vi "State Logger.vi"() -> ()   [LabVIEW 2011, in "Messenging.lvlib" / "State Logger.lvclass"]
uses:
  State Logger.lvclass
  Interprocess Messenger/TextVarientMessage/MSG.lvclass
  Parallel Process.lvclass
  Interprocess Messenger/TextVarientMessage/Write (no data).vi
  Interprocess Messenger/EventMessenger/EventMessenger.lvclass
  Messsage Logger/MessageLoggerMessage/MessageLoggerMessage.lvclass
  <vilib>/Utility/error.llb/DialogType.ctl
  Messsage Logger/Message Logger.lvclass
  Interprocess Messenger/Send/Send.lvclass
panel:
  in  "Displayed Process":i32(listbox) caption="Sent By:"
  in  "Startup Message":refnum<class "MSG.lvclass">
  out "Table":string[][](table)
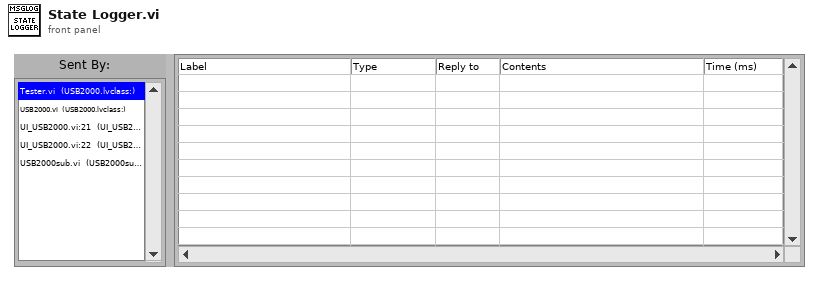
[diagram p1: front panel]
types:
  T1 = enum32{"invalid app kind", "Development System", "Run Time System", "Student Edition", "Embedded LabVIEW", "Evaluation", "Custom"}
  T2 = enum32{"Invalid", "Standard", "Closed", "Hidden", "Minimized", "Maximized"}
  T3 = cluster{"Core":cluster{"Current VI Reference":refnum<vi>, "Close Panel on Exit?":bool}, "New":cluster{"Message":refnum<class "MSG.lvclass">, "MessageTime":u32, "ProcessIndex":i32}, "事件注册引用句柄":refnum<event-registration>, "Processes":string[], "States":cluster{"Table":string[][]}[], "T0":u32}
  T4 = typedef "DialogType.ctl" = u16
  T5 = cluster{"Message":refnum<class "MSG.lvclass">, "MessageTime":u32, "ProcessIndex":i32}
  T6 = cluster{"Current VI Reference":refnum<vi>, "Close Panel on Exit?":bool}
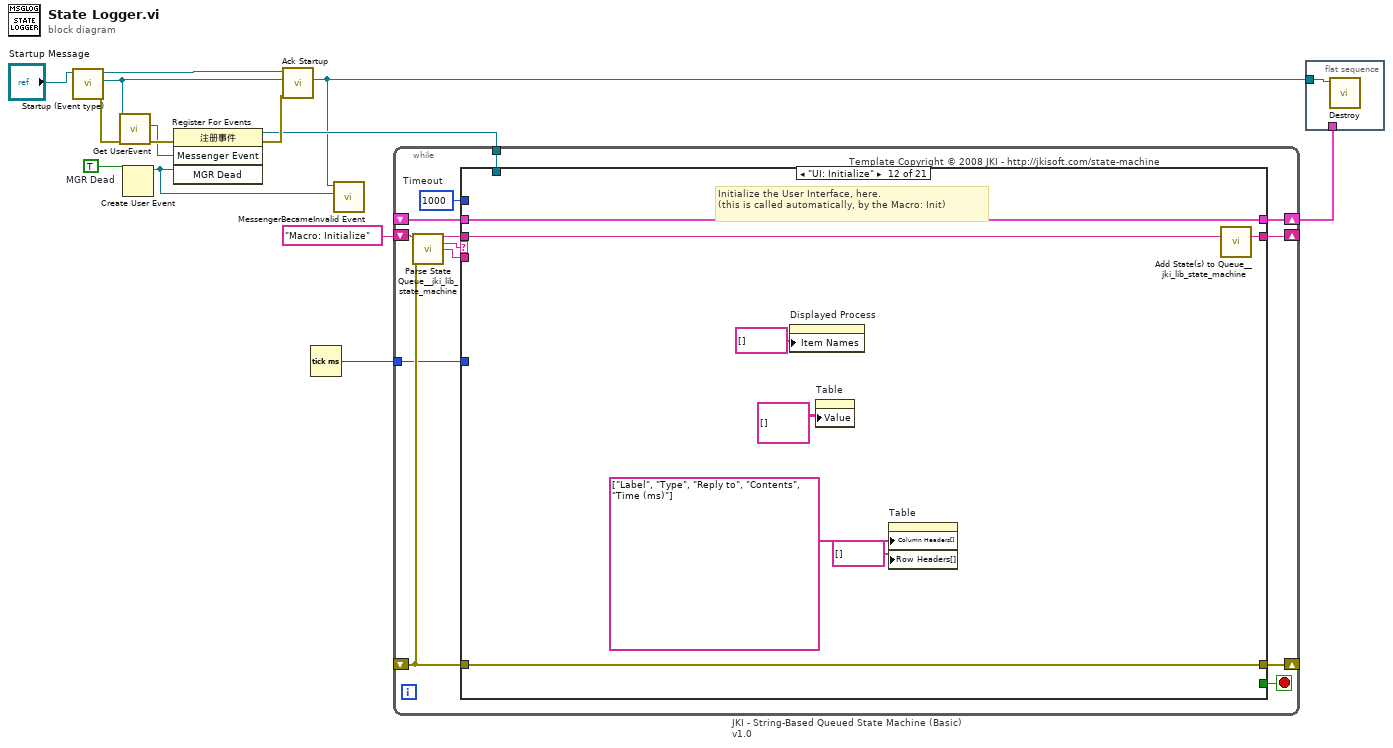
[diagram p0: block diagram]
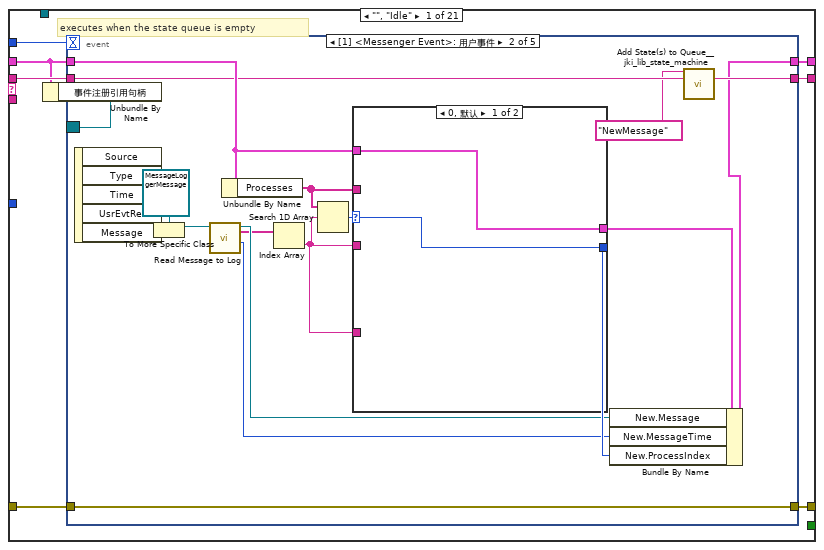
[diagram p2: hidden frame]
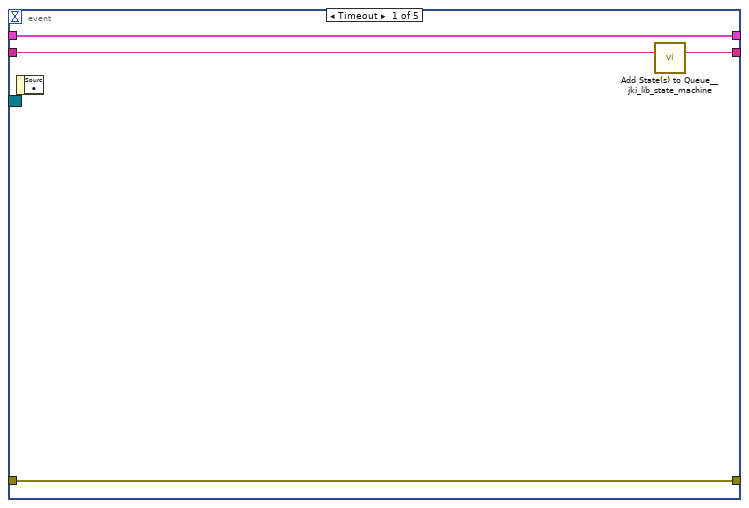
[diagram p3: hidden frame]
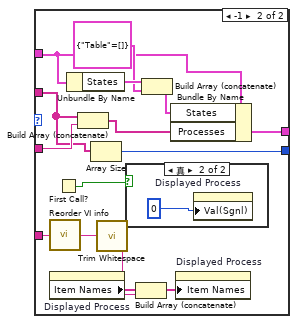
[diagram p4: hidden frame]
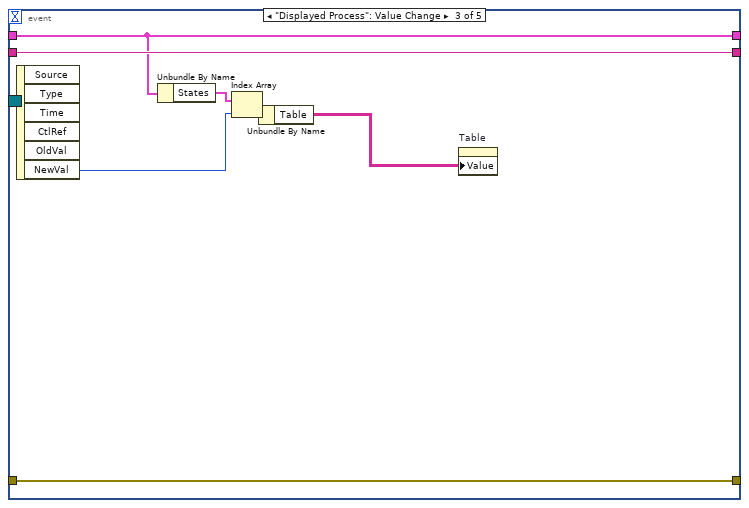
[diagram p6: hidden frame]
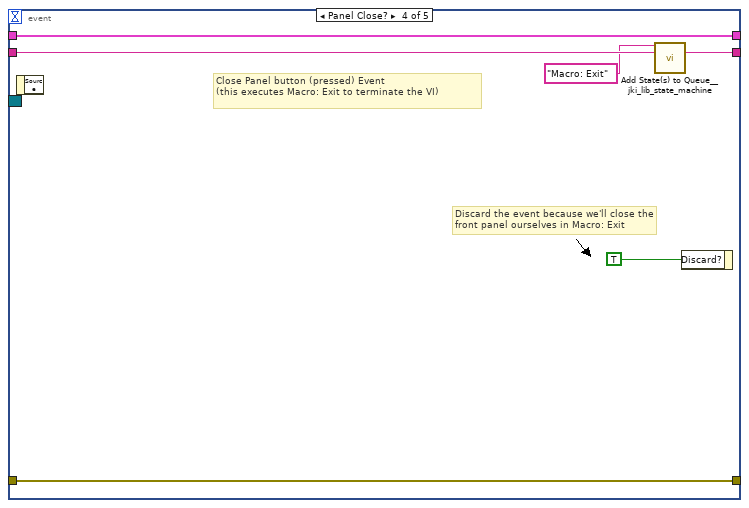
[diagram p7: hidden frame]
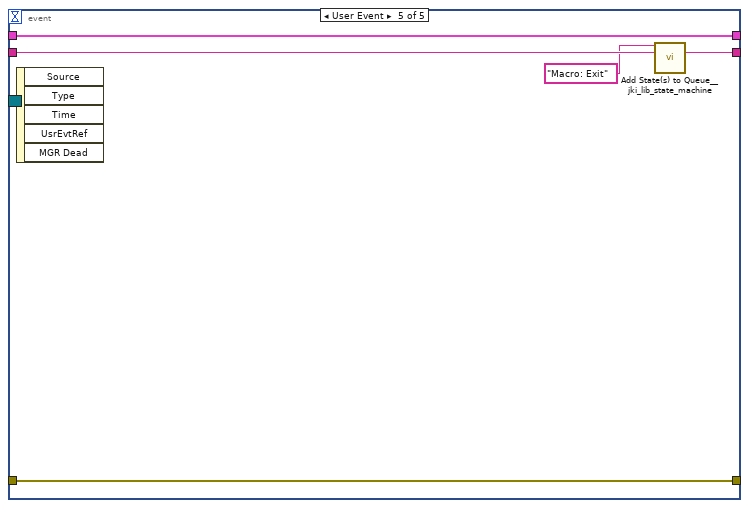
[diagram p8: hidden frame]
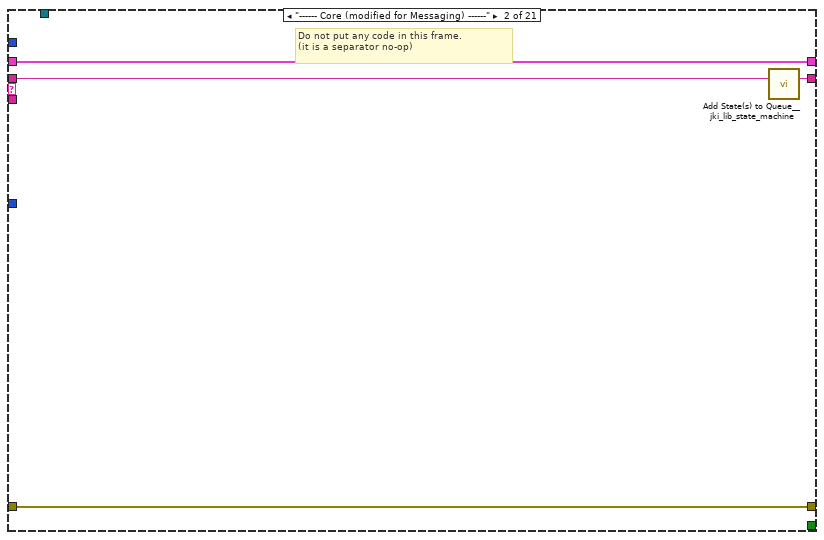
[diagram p9: hidden frame]
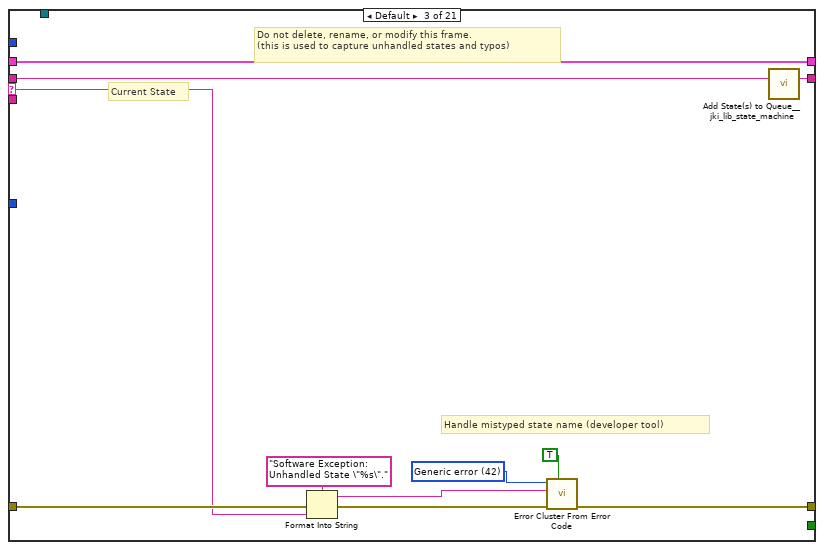
[diagram p10: hidden frame]
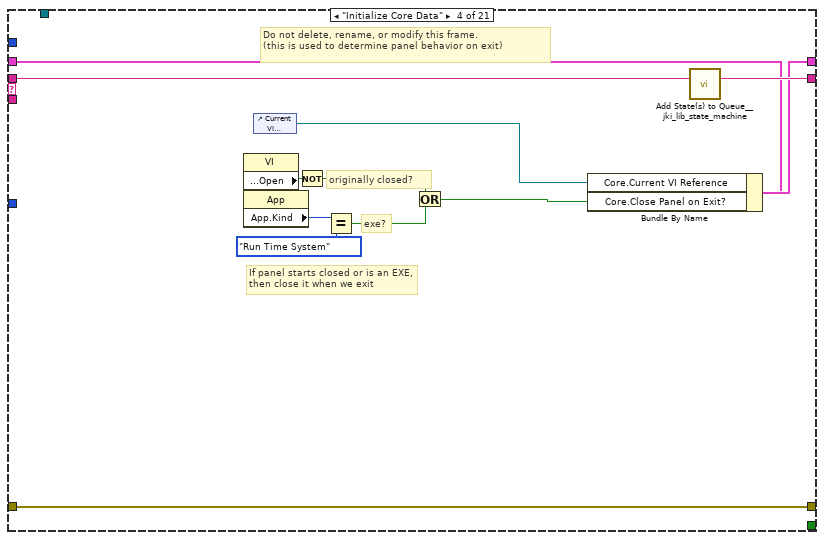
[diagram p11: hidden frame]
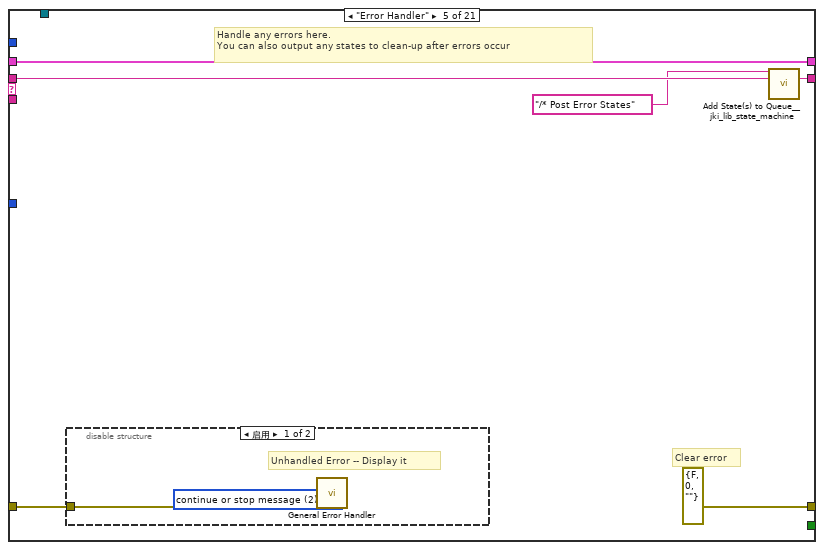
[diagram p12: hidden frame]
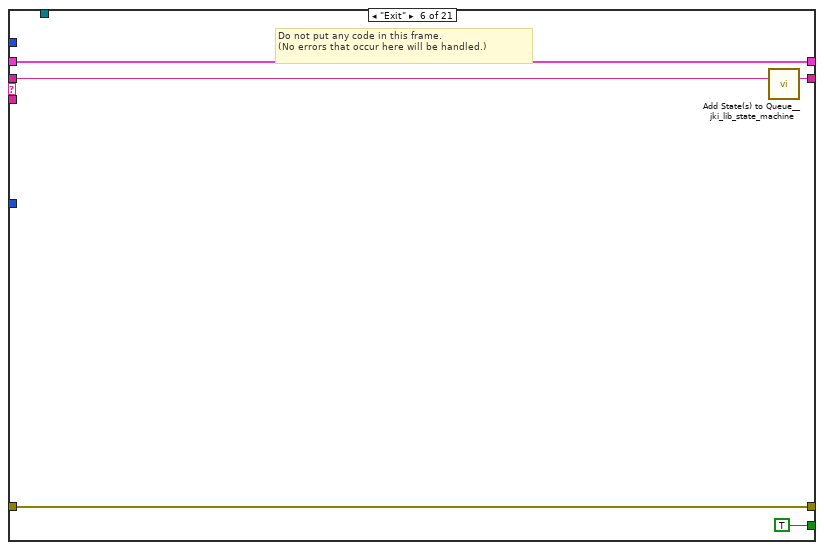
[diagram p14: hidden frame]
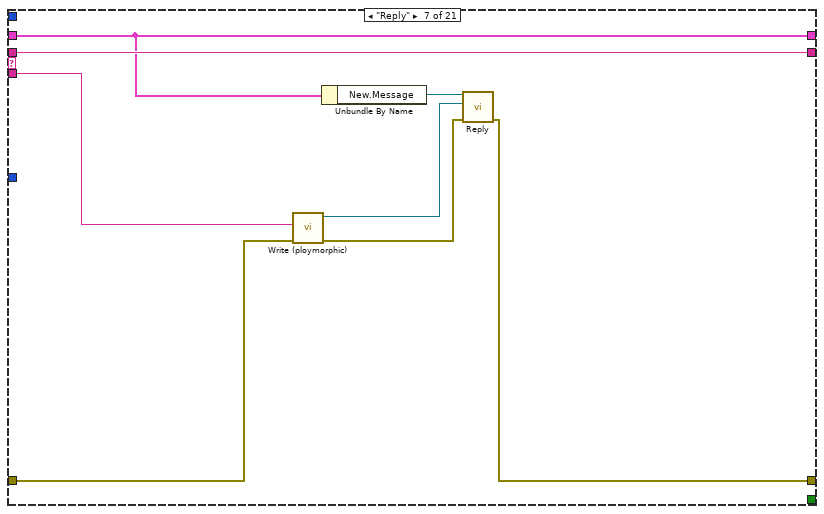
[diagram p15: hidden frame]
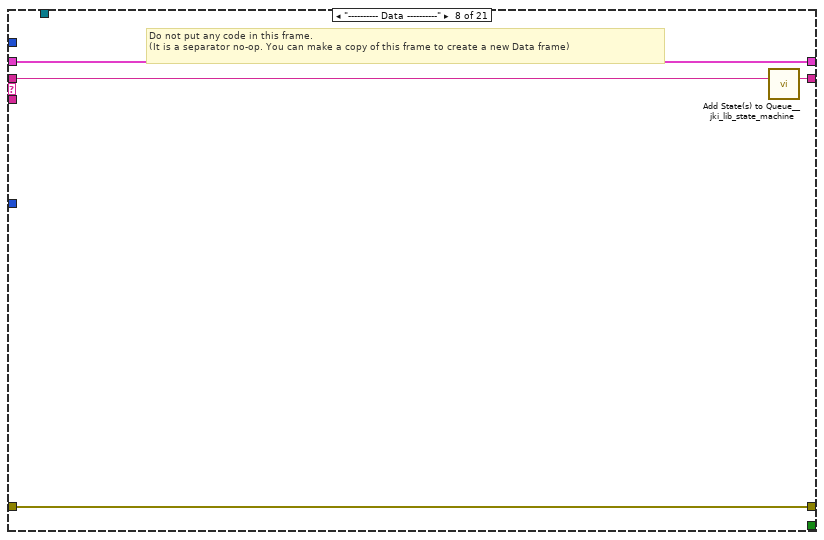
[diagram p16: hidden frame]
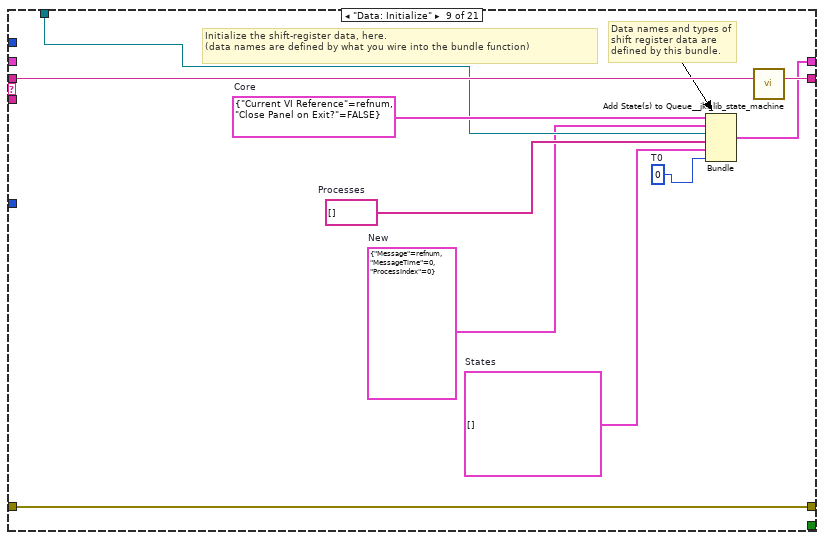
[diagram p17: hidden frame]
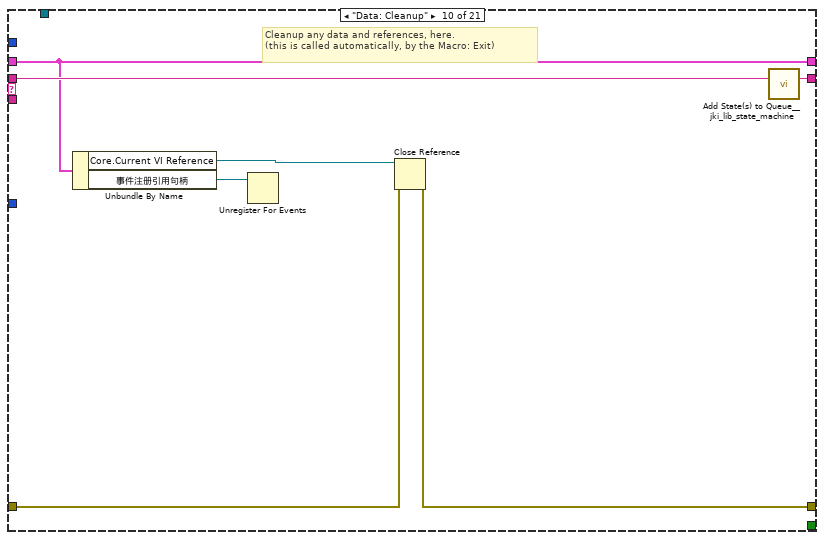
[diagram p18: hidden frame]
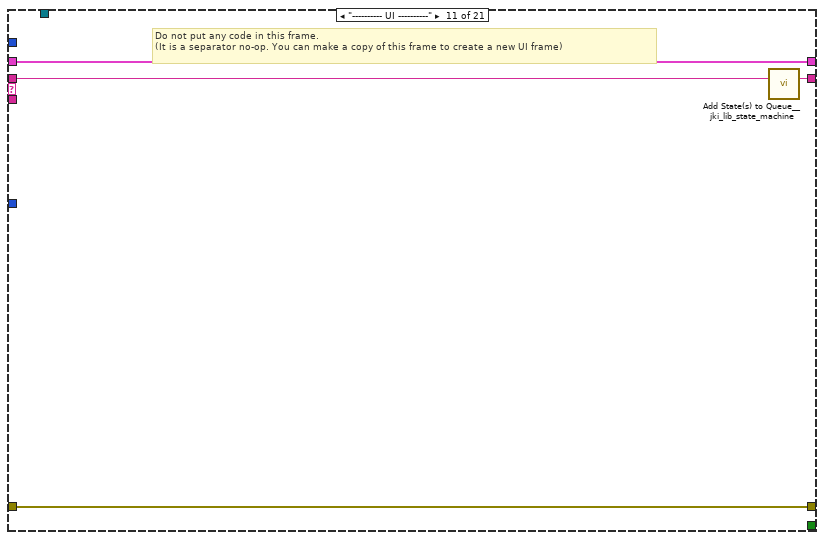
[diagram p19: hidden frame]
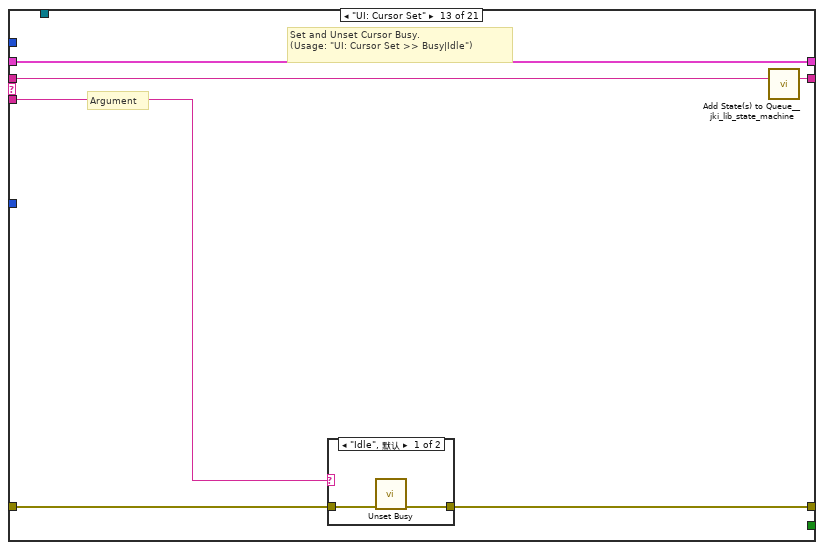
[diagram p20: hidden frame]
diagram:
  w8 = TRUE  # MGR Dead
  n1 = call "Startup (Event type).vi"("Startup Message"="Startup Message") -> ("error out"=w11:errorcluster, "Command Messenger out"=w13:refnum<class "EventMessenger.lvclass">, "Starup Message"=w12:refnum<class "MSG.lvclass">)  [unwired: 2 in, 6 out]
  n2 = call-dynamic "Get UserEvent.vi"("error in"=w11, "EventMessenger"=w13) -> ("error out"=w10:errorcluster, "Messenger Event"=w9:refnum<user-event>)  [unwired: 8 out]
  n3 = Create User Event(user event datatype=w8) -> (user event=w6:refnum<user-event>)  [unwired: 1 in, 1 out]
  n4 = register-events(error in=w10, w9, w6) -> (reference out=w5:refnum<event-registration>, error out=w7:errorcluster)  [unwired: 1 in]
  n5 = call "Ack Startup.vi"("error in"=w7, "Command Messenger"=w13, "Starup Message"=w12) -> ("Command Messenger"=w4:refnum<class "EventMessenger.lvclass">)  [unwired: 3 in, 5 out]
  n6 = Tick Count (ms)() -> (millisecond timer value=w1:u32)
  n7 = call "MessengerBecameInvalid Event.vi"("MGR became Invalid"=w6, "Messenger"=w4) -> ()  [unwired: 1 in, 9 out]
  n8 = while "JKI - String-Based Queued State Machine (Basic) v1.0" {
    shift-right: [w20] -> w3
    shift-left: _ -> [w19]
    shift-right: [w23] -> _
    shift-left: _ -> [w17]
    shift-right: [w22] -> _
    shift-left: "Macro: Initialize" -> [w24]
    tunnel: w5 -> [w16]
    tunnel: w1 -> [w15]
    stop <- w21 stop-if-true
    w18 = 1000  # Timeout
    # "Template Copyright © 2008 JKI - http://jkisoft.com/state-machine"
    n9 = call <vilib>:"Parse State Queue__jki_lib_state_machine.vi"("State Queue"=w24, "Error In (no error)"=w17) -> ("Remaining States"=w26:string, "Current State"=w27:string, "Arguments"=w25:string)  [unwired: 1 in, 10 out]
    n10 = case shown="\"UI: Initialize\"" w27 {
      selector: w27 -> [_ _ w100 _ _ _ _ _ _ _ _ _ _ _ _ _ _ _ _ _ _]
      tunnel: w26 -> [w35 w96 w103 w119 w125 w132 w140 w144 w154 w161 w165 w173 w179 w190 w214 w219 w224 w234 w238 w242 w252]
      tunnel: w25 -> [_ _ _ _ _ _ w133 _ _ _ _ _ w174 w184 _ _ _ _ _ _ _]
      tunnel: w19 -> [w29 w93 w99 w110 w121 w130 w136 w141 _ w156 w162 w171 w177 w186 w213 w216 w220 w225 w235 w241 w248]
      tunnel: [w33 w94 w97 w116 errorcluster {"status"=FALSE, "code"=0, "source"=""} ("error out") w129 w134 w142 w151 w157 w163 w170 w175 w187 w215 w217 w222 w232 w236 w243 w273] -> w23
      tunnel: w17 -> [w32 w94 w104 w116 w120 w129 w135 w142 w151 w158 w163 w170 w176 w188 w215 w217 w222 w232 w236 w243 w273]
      tunnel: [w34 w95 w102 w118 w124 w131 w140 w143 w153 w160 w164 w172 w178 w189 w214 w218 w223 w233 w237 w242 w252] -> w22
      tunnel: [_ _ _ _ _ TRUE _ _ _ _ _ _ _ _ _ _ _ _ _ _ _] -> w21
      tunnel: [w31 w93 w99 w117 w121 w130 w136 w141 w152 w156 w162 w171 w177 w186 w213 w216 w220 w225 w235 w240 w256] -> w20
      tunnel: w18 -> [w30 _ _ _ _ _ _ _ _ _ _ _ _ _ _ _ _ _ _ _ _]
      tunnel: w16 -> [_ _ _ _ _ _ _ _ w149 _ _ _ _ _ _ _ _ _ _ _ _]
      tunnel: w15 -> [_ _ _ _ _ _ _ _ _ _ _ _ _ _ _ _ _ _ _ w239 _]
      frame "", "Idle" {
        # "executes when the state queue is empty"
        n11 = Unbundle By Name(w29) -> ("事件注册引用句柄"=w28:refnum<event-registration>)
        n12 = event shown="[1] <Messenger Event>: 用户事件" {
          selector: w28 -> [_ _ _ _ _]
          dyn-events: _ -> [_ _ _ _ _]
          timeout: w30 -> [_ _ _ _ _]
          tunnel: w35 -> [w39 w49 w81 w87 w92]
          tunnel: [w38 w56 w81 w86 w91] -> w34
          tunnel: w29 -> [w36 w51 w79 w84 w89]
          tunnel: [w37 w52 w80 w85 w90] -> w33
          tunnel: w32 -> [w37 w52 w80 w85 w90]
          tunnel: [w36 w50 w79 w84 w89] -> w31
          event Timeout {
            n13 = event-data() -> ()  [unwired: 2 out]
            n14 = call <vilib>:"Add State(s) to Queue__jki_lib_state_machine.vi"("State(s) in (\"\")"=w39) -> ("States Out"=w38:string)  [unwired: 2 in, 12 out]
          }
          event User Event {
            n15 = event-data() -> ("Message"=w53:refnum<class "MSG.lvclass">)  [unwired: 5 out]
            n16 = To More Specific Class(target class=refnum<class "MessageLoggerMessage.lvclass"> refnum ("Parallel Process.lvlib:MessageLoggerMessage.lvclass"), reference=w53) -> (specific class reference=w55:refnum<class "MessageLoggerMessage.lvclass">)  [unwired: 1 in, 1 out]
            n17 = call "Read Message to Log.vi"("MessageLoggerMessage.lvclass in"=w55) -> ("millisecond timer"=w44:u32, "call chain"=w41:string[], "Messenging.lvlib:Interprocess Message"=w43:refnum<class "MSG.lvclass">)  [unwired: 1 in, 7 out]
            n18 = Unbundle By Name(w51) -> ("Processes"=w46:string[])
            n19 = Index Array(array=w41) -> (element=w40:string)  [unwired: 1 in]
            n20 = Search 1D Array(1D array=w46, element=w40) -> (index of element=w47:i32)  [unwired: 1 out]
            n21 = case shown="0, 默认" w47 {
              selector: w47 -> [w58 _]
              tunnel: [w57 w73] -> w48
              tunnel: w51 -> [w57 w59]
              tunnel: w46 -> [_ w64]
              tunnel: w40 -> [_ w72]
              tunnel: [w58 w70] -> w45
              tunnel: w40 -> [_ w69]
              frame 0, Default {
              }
              frame -1 {
                n22 = call "Reorder VI info.vi"("chain"=w69) -> ("Reorderded"=w65:string)
                n23 = property on="Displayed Process" class="LstBox (严格)"() -> ("Item Names"=w68:string[])  [unwired: 2 in, 2 out]
                n24 = First Call?() -> (First Call?: T/F=w60:bool)
                n25 = Unbundle By Name(w59) -> ("States"=w63:cluster{"Table":string[][]}[])
                n26 = Build Array (concatenate)(w64, w72) -> (w71:string[])
                n27 = Array Size(array=w64) -> (size(s)=w70:i32)
                n28 = call <vilib>:"Trim Whitespace.vi"("string"=w65) -> ("trimmed string"=w66:string)  [unwired: 1 in]
                n29 = case shown="真" w60 {
                  frame False {
                  }
                  frame True {
                    n30 = property on="Displayed Process" class="LstBox (严格)"("Val(Sgnl)"=0 ("Value (Signaling)")) -> ()  [unwired: 2 in, 2 out]
                  }
                }
                n31 = Build Array (concatenate)(w68, w66) -> (w67:string[])
                n32 = Build Array (concatenate)(w63, cluster{"Table":string[][]} {"Table"=[]} ("element")) -> (w61:cluster{"Table":string[][]}[])
                n33 = Bundle By Name(cluster=w59, "States"=w61, "Processes"=w71) -> (w73:T3)
                n34 = property on="Displayed Process" class="LstBox (严格)"("Item Names"=w67) -> ()  [unwired: 2 in, 2 out]
              }
            }
            n35 = Bundle By Name(cluster=w48, "New.Message"=w43, "New.MessageTime"=w44, "New.ProcessIndex"=w45) -> (w50:T3)
            n36 = call <vilib>:"Add State(s) to Queue__jki_lib_state_machine.vi"("State(s) in Front (\"\")"="NewMessage" ("State(s) in Front (\"\")"), "State(s) in (\"\")"=w49) -> ("States Out"=w56:string)  [unwired: 1 in, 12 out]
          }
          event "Displayed Process": Value Change {
            n37 = event-data() -> ("NewVal"=w77:i32)  [unwired: 6 out]
            n38 = Unbundle By Name(w79) -> ("States"=w78:cluster{"Table":string[][]}[])
            n39 = Index Array(array=w78, index=w77) -> (element=w76:cluster{"Table":string[][]})
            n40 = Unbundle By Name(w76) -> ("Table"=w75:string[][])
            n41 = property on="Table" class="Tbl (严格)"("Value"=w75) -> ()  [unwired: 2 in, 2 out]
          }
          event Panel Close? {
            # "Discard the event because we'll close the front panel ourselves in Macro: Exit"
            # "Close Panel button (pressed) Event\n(this executes Macro: Exit to terminate the VI)"
            n42 = event-data() -> ()  [unwired: 2 out]
            n43 = call <vilib>:"Add State(s) to Queue__jki_lib_state_machine.vi"("State(s) in Front (\"\")"="Macro: Exit", "State(s) in (\"\")"=w87) -> ("States Out"=w86:string)  [unwired: 1 in, 12 out]
            n44 = event-data("Discard?"=TRUE) -> ()  [unwired: 1 in, 1 out]
          }
          event User Event {
            n45 = event-data() -> ()  [unwired: 6 out]
            n46 = call <vilib>:"Add State(s) to Queue__jki_lib_state_machine.vi"("State(s) in Front (\"\")"="Macro: Exit", "State(s) in (\"\")"=w92) -> ("States Out"=w91:string)  [unwired: 1 in, 12 out]
          }
        }
      }
      frame "------ Core (modified for Messaging) ------" {
        # "Do not put any code in this frame.\n(it is a separator no-op)"
        n47 = call <vilib>:"Add State(s) to Queue__jki_lib_state_machine.vi"("State(s) in (\"\")"=w96) -> ("States Out"=w95:string)  [unwired: 2 in, 12 out]
      }
      frame Default {
        w106 = 42 items=["No error", "Argument error", "Memory is full", "Out of zone", "End of file", "File already open", "Generic file I/O error", "File not found", "File permission error", "Disk is full", "Duplicate path", "Too many files open", "System feature not enabled", "Resource file not found", "Cannot add resource", "Resource not found", "Image not found", "Image memory error", "Pen does not exist", "Config type invalid", "Config token not found", "Config parse error", "Config memory error", "Bad external code format", "Bad external code offset", "External code not present", "Null window", "Destroy window error", "Null menu", "Print aborted", "Bad print record", "Print driver error", "Windows error during printing", "Memory error during printing", "Print dialog error", "Generic print error", "Invalid device refnum", "Device not found", "Device parameter error", "Device unit error", "Cannot open device", "Device call aborted", "Generic error", "Cancelled by user", "Object ID too low", "Object ID too high", "Object not in heap", "Unknown heap", "Unknown object (invalid DefProc)", "Unknown object (DefProc not in table)", "Message out of range", "Invalid (null) method", "Unknown message", "Manager call not supported", "Bad address", "Network operation in progress", "Network operation timed out", "Connection is busy", "Network attribute not supported", "Network error", "Address in use", "System out of memory", "Connection aborted", "Connection refused", "Not connected", "Already connected", "Connection closed", "Initialization error (interapplication manager)", "Bad occurrence", "Wait on unbound occurrence handler", "Occurrence queue overflow", "Datalog type conflict", "Unused", "Unrecognized type (interapplication manager)", "Memory corrupt", "Failed to make temporary DLL", "Old CIN version", "Drag socket not found", "Failed to load drop-object", "Failed to register OLE object", "Failed to release OLE object", "Format specifier type mismatch", "Unknown format specifier", "Too few format specifiers", "Too many format specifiers", "Scan failed", "Newer CIN version", "Error converting to variant", "Runtime menu error", "Password tampered", "Variant attribute not found", "Incompatible variant data type", "Event data is not available", "Event Store is not present", "Occurrence is not found", "Event Queue is not created", "Event info is not available", "Refnum passed is NULL", "Error retrieving Class GUID", "Error retrieving CoClass GUID", "Error retrieving TypeLib GUID.", "Bad built application magic bytes.", "Specific driver is different from the specific driver associated with the Logical Name.", "There is no session opened to the class driver.", "Max Error", "MAX - Error with config objects", "MAX - Error loading configuration", "MAX - Group not supported"]
        # "Current State"
        # "Do not delete, rename, or modify this frame.\n(this is used to capture unhandled states and typos)"
        # "Handle mistyped state name (developer tool)"
        n48 = Format Into String(format string="Software Exception: Unhandled State \"%s\"." ("message"), error in=w104, w100) -> (resulting string=w98:string, error out=w105:errorcluster)  [unwired: 1 in]
        n49 = call <vilib>:"Error Cluster From Error Code.vi"("show call chain? (False)"=TRUE, "error in (no error)"=w105, "error message (\"\")"=w98, "error code (0)"=w106) -> ("error out"=w97:errorcluster)  [unwired: 5 out]
        n50 = call <vilib>:"Add State(s) to Queue__jki_lib_state_machine.vi"("State(s) in (\"\")"=w103) -> ("States Out"=w102:string)  [unwired: 2 in, 12 out]
      }
      frame "Initialize Core Data" {
        # "Do not delete, rename, or modify this frame.\n(this is used to determine panel behavior on exit)"
        # "originally closed?"
        # "exe?"
        # "If panel starts closed or is an EXE, then close it when we exit"
        n51 = property class="VI"() -> ("Front Panel.Open"=w115:bool)  [unwired: 2 in, 2 out]
        n52 = property class="App"() -> ("App.Kind"=w114:T1)  [unwired: 2 in, 2 out]
        n53 = control-ref of="Current VI Reference"() -> (w108:refnum<vi>)
        n54 = Not(x=w115) -> (.not. x?=w112:bool)
        n55 = Equal?(x=w114, y=T1."Run Time System" ("Application:Kind")) -> (x = y?=w111:bool)
        n56 = Or(x=w112, y=w111) -> (x .or. y?=w109:bool)
        n57 = Bundle By Name(cluster=w110, "Core.Current VI Reference"=w108, "Core.Close Panel on Exit?"=w109) -> (w117:T3)
        n58 = call <vilib>:"Add State(s) to Queue__jki_lib_state_machine.vi"("State(s) in (\"\")"=w119) -> ("States Out"=w118:string)  [unwired: 2 in, 12 out]
      }
      frame "Error Handler" {
        # "Handle any errors here.\nYou can also output any states to clean-up after errors occur"
        # "Clear error"
        n59 = disable-structure shown="启用" {
          disable-tunnel: w120 -> [w127 _]
          frame Enabled {
            w126 = T4 2 items=["no dialog", "OK message", "continue or stop message", "OK message + warnings", "continue/stop + warnings"] ("type of dialog (OK msg:1)")
            # "Unhandled Error -- Display it"
            n60 = call <vilib>:"General Error Handler.vi"("type of dialog (OK msg:1)"=w126, "error in (no error)"=w127) -> ()  [unwired: 14 out]
          }
          frame Disabled {
          }
        }
        n61 = call <vilib>:"Add State(s) to Queue__jki_lib_state_machine.vi"("State(s) in Front (\"\")"="/* Post Error States", "State(s) in (\"\")"=w125) -> ("States Out"=w124:string)  [unwired: 1 in, 12 out]
      }
      frame "Exit" {
        # "Do not put any code in this frame.\n(No errors that occur here will be handled.)"
        n62 = call <vilib>:"Add State(s) to Queue__jki_lib_state_machine.vi"("State(s) in (\"\")"=w132) -> ("States Out"=w131:string)  [unwired: 2 in, 12 out]
      }
      frame "Reply" {
        n63 = call-poly "Write (ploymorphic).vi"("error in (no error)"=w135, "Label"=w133) -> ("error out"=w137:errorcluster, "Message"=w138:refnum<class "MSG.lvclass">)  [unwired: 8 out]
        n64 = Unbundle By Name(w136) -> ("New.Message"=w139:refnum<class "MSG.lvclass">)
        n65 = call-dynamic "Reply.vi"("error in (no error)"=w137, "Reply"=w138, "Message to Reply to"=w139) -> ("error out"=w134:errorcluster)  [unwired: 8 out]
      }
      frame "---------- Data ----------" {
        # "Do not put any code in this frame.\n(It is a separator no-op. You can make a copy of this frame to create a new Data frame)"
        n66 = call <vilib>:"Add State(s) to Queue__jki_lib_state_machine.vi"("State(s) in (\"\")"=w144) -> ("States Out"=w143:string)  [unwired: 2 in, 12 out]
      }
      frame "Data: Initialize" {
        w146 = cluster{"Table":string[][]}[] []  # States
        w147 = T5 {"Message"=refnum, "MessageTime"=0, "ProcessIndex"=0}  # New
        w145 = u32 0  # T0
        w148 = string[] []  # Processes
        w150 = T6 {"Current VI Reference"=refnum, "Close Panel on Exit?"=FALSE}  # Core
        # "Data names and types of shift register data are defined by this bundle."
        # "Initialize the shift-register data, here.\n(data names are defined by what you wire into the bundle function)"
        n67 = Bundle("Core"=w150, "New"=w147, "事件注册引用句柄"=w149, "Processes"=w148, "States"=w146, "T0"=w145) -> (w152:T3)  [unwired: 1 out]
        n68 = call <vilib>:"Add State(s) to Queue__jki_lib_state_machine.vi"("State(s) in (\"\")"=w154) -> ("States Out"=w153:string)  [unwired: 2 in, 12 out]
      }
      frame "Data: Cleanup" {
        # "Cleanup any data and references, here.\n(this is called automatically, by the Macro: Exit)"
        n69 = Unbundle By Name(w156) -> ("Core.Current VI Reference"=w159:refnum<vi>, "事件注册引用句柄"=w155:refnum<event-registration>)
        n70 = Unregister For Events(event registration refnum=w155) -> ()  [unwired: 1 in, 1 out]
        n71 = Close Reference(reference=w159, error in (no error)=w158) -> (error out=w157:errorcluster)
        n72 = call <vilib>:"Add State(s) to Queue__jki_lib_state_machine.vi"("State(s) in (\"\")"=w161) -> ("States Out"=w160:string)  [unwired: 2 in, 12 out]
      }
      frame "---------- UI ----------" {
        # "Do not put any code in this frame.\n(It is a separator no-op. You can make a copy of this frame to create a new UI frame)"
        n73 = call <vilib>:"Add State(s) to Queue__jki_lib_state_machine.vi"("State(s) in (\"\")"=w165) -> ("States Out"=w164:string)  [unwired: 2 in, 12 out]
      }
      frame "UI: Initialize" {
        # "Initialize the User Interface, here.\n(this is called automatically, by the Macro: Init)"
        n74 = property on="Displayed Process" class="LstBox (严格)"("Item Names"=string[] []) -> ()  [unwired: 2 in, 2 out]
        n75 = property on="Table" class="Tbl (严格)"("Value"=string[][] [] ("Table")) -> ()  [unwired: 2 in, 2 out]
        n76 = property on="Table" class="Tbl (严格)"("Column Headers[]"=string[] ["Label", "Type", "Reply to", "Contents", "Time (ms)"] ("Row Header Strings[]"), "Row Headers[]"=string[] [] ("Row Header Strings[]")) -> ()  [unwired: 2 in, 2 out]
        n77 = call <vilib>:"Add State(s) to Queue__jki_lib_state_machine.vi"("State(s) in (\"\")"=w173) -> ("States Out"=w172:string)  [unwired: 2 in, 12 out]
      }
      frame "UI: Cursor Set" {
        # "Argument"
        # "Set and Unset Cursor Busy.\n(Usage: \"UI: Cursor Set >> Busy|Idle\")"
        n78 = case shown="\"Idle\", 默认" w174 {
          tunnel: w176 -> [w181 w183]
          tunnel: [w180 w182] -> w175
          frame "Idle", Default {
            n79 = call <vilib>:"Unset Busy.vi"("error in (no error)"=w181) -> ("error out"=w180:errorcluster)  [unwired: 1 in, 9 out]
          }
          frame "Busy" {
            n80 = call <vilib>:"Set Busy.vi"("error in (no error)"=w183) -> ("error out"=w182:errorcluster)  [unwired: 3 in, 7 out]
          }
        }
        n81 = call <vilib>:"Add State(s) to Queue__jki_lib_state_machine.vi"("State(s) in (\"\")"=w179) -> ("States Out"=w178:string)  [unwired: 2 in, 12 out]
      }
      frame "UI: Front Panel State" {
        # "Argument"
        # "Set Front Panel Open or Closed\n(Usage: \"UI: Front Panel State >> Open|Close\")"
        n82 = Unbundle By Name(w186) -> ("Core.Current VI Reference"=w185:refnum<vi>)
        n83 = case shown="\"Open\", 默认" w184 {
          tunnel: w188 -> [w194 w207]
          tunnel: [w196 w208] -> w187
          tunnel: w185 -> [w195 w205]
          frame "Open", Default {
            n84 = property class="VI"(reference=w195, error in=w194) -> (reference out=w192:refnum<vi>, error out=w193:errorcluster, "Front Panel.Open"=w191:bool)
            n85 = case shown="假" w191 {
              tunnel: [w199 w202] -> w196
              tunnel: w193 -> [w198 w202]
              tunnel: w192 -> [w197 _]
              frame False {
                n86 = invoke class="VI" method="FP.Open"(reference=w197, error in=w198, "Activate"=TRUE, "State"=T2."Standard") -> (error out=w199:errorcluster)  [unwired: 1 in, 4 out]
              }
              frame True {
              }
            }
          }
          frame "Close" {
            n87 = property class="VI"(reference=w205, error in=w207) -> (reference out=w204:refnum<vi>, error out=w206:errorcluster, "Front Panel.Open"=w203:bool)
            n88 = case shown="真" w203 {
              tunnel: [w209 w212] -> w208
              tunnel: w206 -> [w209 w211]
              tunnel: w204 -> [_ w210]
              frame False {
              }
              frame True {
                n89 = invoke class="VI" method="FP.Close"(reference=w210, error in=w211) -> (error out=w212:errorcluster)  [unwired: 1 in, 2 out]
              }
            }
          }
        }
        n90 = call <vilib>:"Add State(s) to Queue__jki_lib_state_machine.vi"("State(s) in (\"\")"=w190) -> ("States Out"=w189:string)  [unwired: 2 in, 12 out]
      }
      frame "UI: ProcessSelect" {
        n91 = Unbundle By Name(w213) -> ()  [unwired: 1 out]
      }
      frame "---------- Macro ----------" {
        # "Do not put any code in this frame.\n(It is a separator no-op. You can make a copy of this frame to create a new Macro frame)"
        n92 = call <vilib>:"Add State(s) to Queue__jki_lib_state_machine.vi"("State(s) in (\"\")"=w219) -> ("States Out"=w218:string)  [unwired: 2 in, 12 out]
      }
      frame "Macro: Initialize" {
        w221 = "Data: Initialize\nInitialize Core Data\nUI: Initialize\nInitialize\n// UI: Front Panel State >> Open"  # Data: Initialize Initialize Core Data UI: Initialize Initialize // UI: Front Panel State >> Open
        # "Initialization Macro\n(This is called once, when the VI starts)"
        n93 = call <vilib>:"Add State(s) to Queue__jki_lib_state_machine.vi"("State(s) in Front (\"\")"=w221, "State(s) in (\"\")"=w224) -> ("States Out"=w223:string)  [unwired: 1 in, 12 out]
      }
      frame "Macro: Exit" {
        # "Exit Macro\n(This is called once, when the VI exits)"
        n94 = Unbundle By Name(w225) -> ("Core.Close Panel on Exit?"=w231:bool)
        n95 = Select(t="//UI: Front Panel State >> Close", s=w231, f="") -> (s? t:f=w228:string)
        n96 = call <vilib>:"Add State(s) to Queue__jki_lib_state_machine.vi"("State(s) in (\"\")"=w228, "State(s) at Back (\"\")"="\nData: Cleanup\nExit") -> ("States Out"=w226:string)  [unwired: 1 in, 12 out]
        n97 = call <vilib>:"Add State(s) to Queue__jki_lib_state_machine.vi"("State(s) in Front (\"\")"=w226, "State(s) in (\"\")"=w234) -> ("States Out"=w233:string)  [unwired: 1 in, 12 out]
      }
      frame "---------- New Category ----------" {
        # "Template Separator\n(You can make a copy of, or modify, this frame)"
        n98 = call <vilib>:"Add State(s) to Queue__jki_lib_state_machine.vi"("State(s) in (\"\")"=w238) -> ("States Out"=w237:string)  [unwired: 2 in, 12 out]
      }
      frame "Initialize" {
        n99 = Bundle By Name(cluster=w241, "T0"=w239) -> (w240:T3)
      }
      frame "NewMessage" {
        n100 = Unbundle By Name(w248) -> ("States"=w259:cluster{"Table":string[][]}[], "New.ProcessIndex"=w253:i32)
        n101 = Unbundle By Name(w248) -> ("New.Message"=w265:refnum<class "MSG.lvclass">)
        n102 = Unbundle By Name(w248) -> ("New.MessageTime"=w247:u32, "T0"=w244:u32)
        n103 = call-dynamic "Read Label.vi"("Message"=w265) -> ("Label"=w264:string, "Message"=w266:refnum<class "MSG.lvclass">)  [unwired: 1 in, 8 out]
        n104 = Index Array(array=w259, index=w253) -> (element=w258:cluster{"Table":string[][]})
        n105 = Equal?(x="Displayed Process", y=w253) -> (x = y?=w251:bool)
        n106 = call-dynamic "Read Reply Messenger.vi"("Messege"=w266) -> ("Reply to..."=w271:refnum<class "Send.lvclass">, "Message"=w270:refnum<class "MSG.lvclass">)  [unwired: 1 in, 8 out]
        n107 = Unbundle By Name(w258) -> ("Table"=w260:string[][])
        n108 = Subtract(x=w247, y=w244) -> (x-y=w245:u32)
        n109 = call-dynamic "Message Class.vi"("Message"=w270) -> ("Message Class"=w267:string, "Message"=w268:refnum<class "MSG.lvclass">)  [unwired: 1 in, 8 out]
        n110 = call-dynamic "Text Description.vi"("Send in"=w271) -> ("Description"=w272:string)  [unwired: 10 out]
        n111 = Index Array(array=w260, index (col)=0 ("index (row)")) -> (element=w261:string[])  [unwired: 1 in]
        n112 = call-dynamic "Contents Summary Text.vi"("Message"=w268) -> ("Contents Summary Text"=w269:string)  [unwired: 10 out]
        n113 = Number To Decimal String(number=w245) -> (decimal integer string=w246:string)  [unwired: 1 out]
        n114 = Search 1D Array(1D array=w261, element=w264) -> (index of element=w263:i32)  [unwired: 1 out]
        n115 = Build Array(w264, w267, w272, w269, w246) -> (w262:string[])
        n116 = case shown="0, 默认" w263 {
          selector: w263 -> [w276 _]
          tunnel: w262 -> [w278 w279]
          tunnel: w260 -> [w277 w281]
          tunnel: [w275 w280] -> w250
          frame 0, Default {
            n117 = Replace Array Subset(array=w277, new element=w278, index (row)=w276) -> (w275:string[][])  [unwired: 1 in]
          }
          frame -1 {
            n118 = Build Array (concatenate)(w281, w279) -> (w280:string[][])
          }
        }
        n119 = Bundle By Name(cluster=w258, "Table"=w250) -> (w257:cluster{"Table":string[][]})
        n120 = case shown="真" w251 {
          tunnel: w250 -> [_ w274]
          frame False {
          }
          frame True {
            "Table" <- w274
          }
        }
        n121 = Replace Array Subset(array=w259, new element=w257, index=w253) -> (w255:cluster{"Table":string[][]}[])
        n122 = Bundle By Name(cluster=w248, "States"=w255) -> (w256:T3)
      }
    }
  }
  n123 = flat-sequence {
    tunnel: w4 -> [w282]
    tunnel: w3 -> [_]
    frame #0 {
      n124 = call-dynamic "Destroy.vi"("EventMessenger in"=w282) -> ()  [unwired: 1 in, 10 out]
    }
  }
